vi "LV-Term UI.vi"(11 "LV-Term App In":refnum<class "LV-Term App.lvclass">) -> (3 "LV-Term App":refnum<class "LV-Term App.lvclass">)   [LabVIEW 2020, in "LV-Term.lvlib" / "LV-Term App.lvclass"]
uses:
  LV-Term App.lvclass
  UI State.ctl
  LV-Term App.lvclass/LV-Term App.ctl
  <vilib>/IlluminatedG/IG Terminal/Key Event Data.ctl
  <vilib>/event_ctls.llb/eventvkey.ctl
  <vilib>/IlluminatedG/IG Terminal/Terminal/Terminal.lvclass
  C:/Program Files (x86)/National Instruments/LabVIEW 2020/vi.lib/IlluminatedG/IG OOPanel/OOPanel/Panel/Panel.lvclass
  <vilib>/IlluminatedG/lv-stream/Connection/Connection.lvclass
  <vilib>/IlluminatedG/IG OOPanel/OOPanel/Manager/Manager.lvclass
  <vilib>/IlluminatedG/IG Terminal/Terminal.lvlib
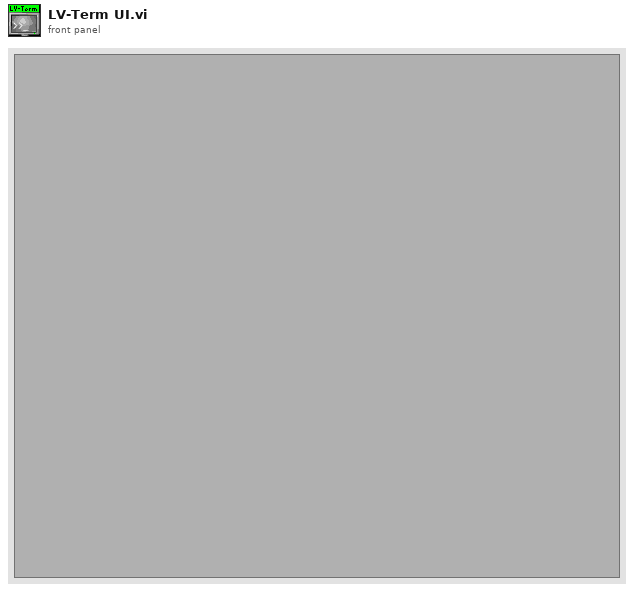
[diagram p1: front panel]
types:
  T1 = typedef "LV-Term.lvlib/LV-Term App.lvclass/UI State.ctl" = enum16{"Init", "Run", "Close"}
  T2 = typedef "Terminal.lvlib/Key Event Data.ctl" = cluster{"Char":i16, "VKey":T3, "ScanCode":i16, "Ctrl":bool}
  T3 = typedef "eventvkey.ctl" = enum16{"ASCII", "Enter", "Return", "Shift", "Ctrl", "Alt", "Cmd", "Opt", "Caps", "NumLock", "Clear", "Break", "Up", "Down", "Left", "Right", "Insert", "Delete", "Home", "End", "PageUp", "PageDown", "Escape", "Help", "Pause", "ScrollLock", "F1", "F2", "F3", "F4", "F5", "F6", "F7", "F8", "F9", "F10", "F11", "F12", "F13", "F14", "F15", "F16", "F17", "F18", "F19", "F20", "F21", "F22", "F23", "F24", "Play", "VolumeUp", "VolumeDown", "Mute", "Two Byte Char"}
  T4 = cluster{"Size Event Reg":refnum<event-registration>}
  T5 = typedef "LVRectTypeDef.ctl" = cluster{"Left":i16, "Top":i16, "Right":i16, "Bottom":i16}
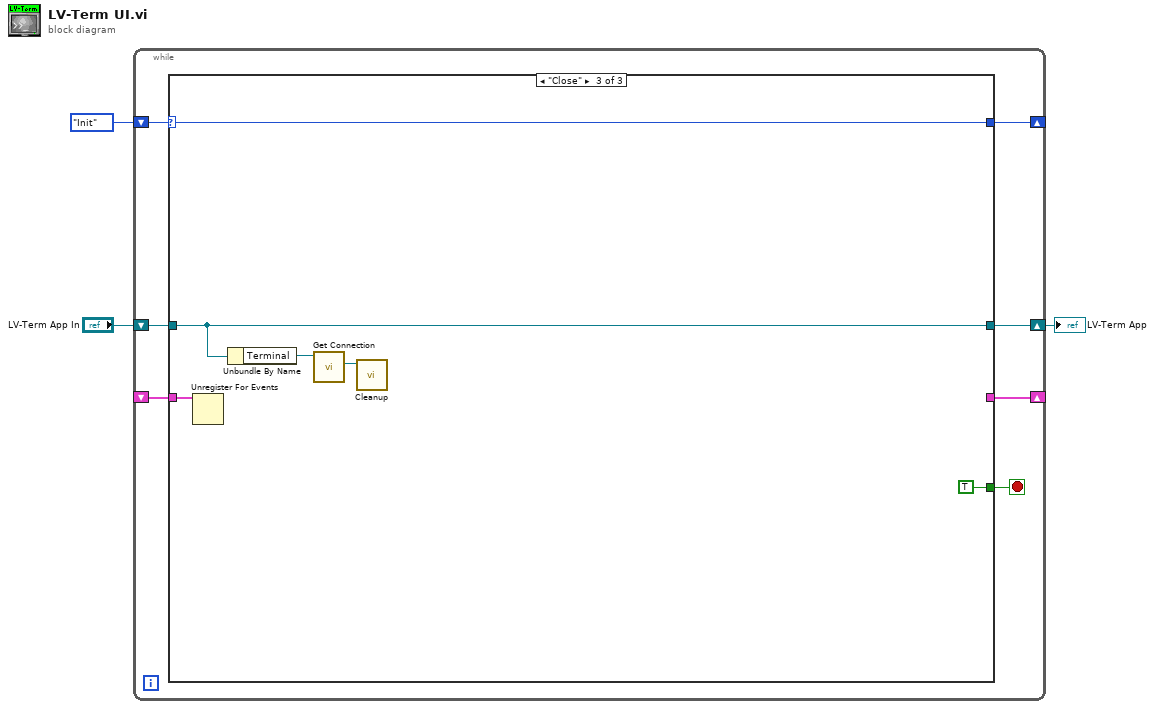
[diagram p0: block diagram]
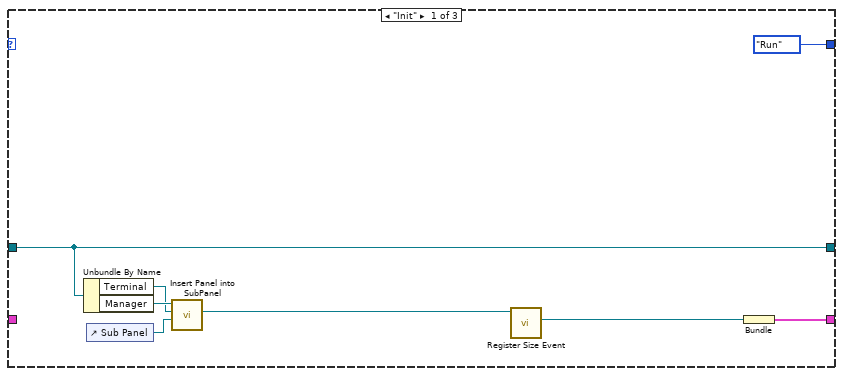
[diagram p2: hidden frame]
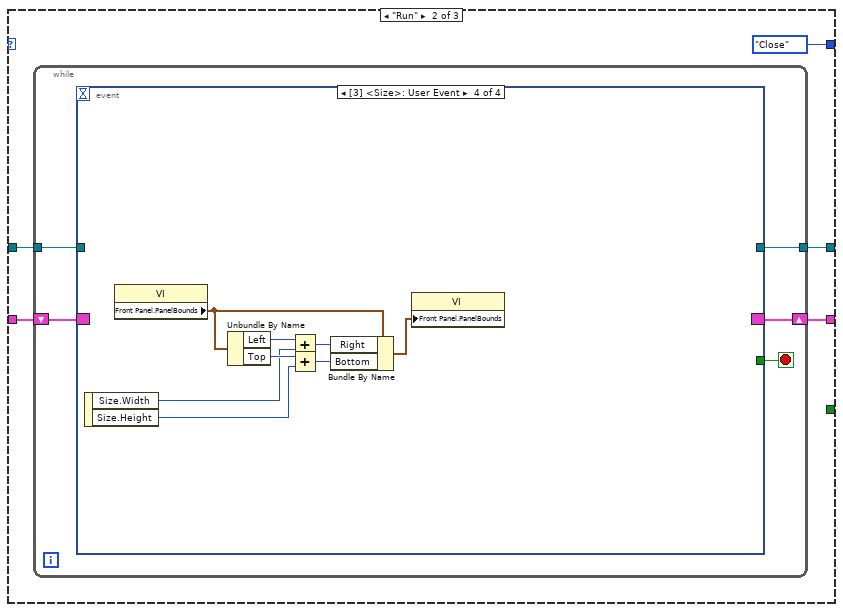
[diagram p3: hidden frame]
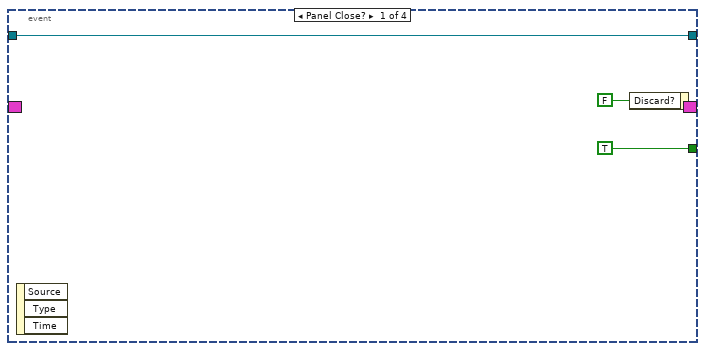
[diagram p4: hidden frame]
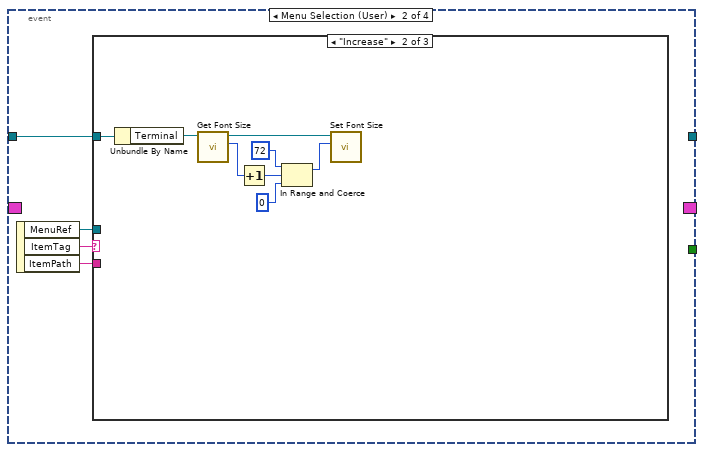
[diagram p5: hidden frame]
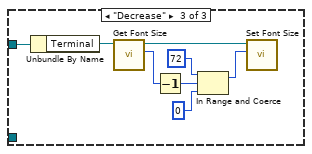
[diagram p7: hidden frame]
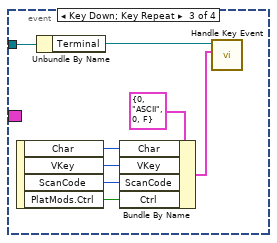
[diagram p8: hidden frame]
diagram:
  n1 = while {
    shift-right: [w9] -> _
    shift-left: UI_State."Init" ("UI State") -> [w10]
    shift-right: [w6] -> w1
    shift-left: "LV-Term App In" -> [w7]
    shift-right: [w5] -> _
    shift-left: _ -> [w4]
    stop <- w8 stop-if-true
    n2 = case shown="\"Close\"" w10 {
      selector: w10 -> [_ _ w72]
      tunnel: [UI_State."Run" ("UI State") UI_State."Close" ("UI State") w72] -> w9
      tunnel: [_ _ TRUE] -> w8
      tunnel: w7 -> [w16 w22 w71]
      tunnel: [w16 w21 w71] -> w6
      tunnel: [w11 w19 _] -> w5
      tunnel: w4 -> [_ w20 w68]
      frame "Init" {
        n3 = Unbundle By Name(w16) -> ("Terminal"=w14:refnum<class "Terminal.lvclass">, "Manager"=w15:refnum<class "Manager.lvclass">)
        n4 = control-ref of="Sub Panel"() -> (w17:refnum<vi>)
        n5 = call <vilib>:"Insert Panel into SubPanel.vi"("SubPanel"=w17, "Panel In"=w14, "Manager in"=w15) -> ("Panel"=w13:refnum<class "Terminal.lvclass">)  [unwired: 6 in, 2 out]
        n6 = call <vilib>:"Register Size Event.vi"("Terminal in"=w13) -> ("Size Event Reg"=w12:refnum<event-registration>)  [unwired: 8 in, 2 out]
        n7 = Bundle("Size Event Reg"=w12) -> (w11:T4)  [unwired: 1 in]
      }
      frame "Run" {
        n8 = while {
          tunnel: w22 -> [w27]
          tunnel: [w26] -> w21
          shift-right: [w24] -> w19
          shift-left: w20 -> [w25]
          stop <- w28 stop-if-true
          n9 = event shown="[3] <Size>: User Event" {
            selector: w25 -> [_ _ _ _]
            dyn-events: [_ _ _ _] -> w24
            timeout: _ -> [_ _ _ _]
            tunnel: [TRUE ("Discard?") _ _ _] -> w28
            tunnel: w27 -> [w29 w32 w59 _]
            tunnel: [w29 _ _ _] -> w26
            event Panel Close? {
              n10 = event-data() -> ()  [unwired: 1 in, 3 out]
              n11 = event-data("Discard?"=FALSE) -> ()  [unwired: 1 in, 1 out]
            }
            event Menu Selection (User) {
              n12 = event-data() -> ("MenuRef"=w34:refnum<k9>, "ItemTag"=w35:string, "ItemPath"=w33:string)  [unwired: 1 in]
              n13 = case shown="\"Increase\"" w35 {
                tunnel: w34 -> [_ _ _]
                tunnel: w33 -> [_ _ _]
                tunnel: w32 -> [_ w36 w51]
                frame Default {
                }
                frame "Increase" {
                  n14 = Unbundle By Name(w36) -> ("Terminal"=w43:refnum<class "Terminal.lvclass">)
                  n15 = call <vilib>:"Get Font Size.vi"("Terminal in"=w43) -> ("Font Size"=w42:i16, "Terminal out"=w38:refnum<class "Terminal.lvclass">)  [unwired: 8 in, 1 out]
                  n16 = Increment(x=w42) -> (x+1=w41:i16)
                  n17 = In Range and Coerce(upper limit=i16 72, x=w41, lower limit=i16 0) -> (coerced(x)=w37:i16)  [unwired: 1 out]
                  n18 = call <vilib>:"Set Font Size.vi"("Font Size"=w37, "Terminal in"=w38) -> ()  [unwired: 8 in, 2 out]
                }
                frame "Decrease" {
                  n19 = Unbundle By Name(w51) -> ("Terminal"=w50:refnum<class "Terminal.lvclass">)
                  n20 = call <vilib>:"Get Font Size.vi"("Terminal in"=w50) -> ("Font Size"=w49:i16, "Terminal out"=w45:refnum<class "Terminal.lvclass">)  [unwired: 8 in, 1 out]
                  n21 = Decrement(x=w49) -> (x-1=w48:i16)
                  n22 = In Range and Coerce(upper limit=i16 72, x=w48, lower limit=i16 0) -> (coerced(x)=w44:i16)  [unwired: 1 out]
                  n23 = call <vilib>:"Set Font Size.vi"("Font Size"=w44, "Terminal in"=w45) -> ()  [unwired: 8 in, 2 out]
                }
              }
            }
            event Key Down; Key Repeat {
              n24 = event-data() -> ("Char"=w55:i16, "VKey"=w54:T3, "ScanCode"=w53:i16, "PlatMods.Ctrl"=w52:bool)  [unwired: 1 in]
              n25 = Unbundle By Name(w59) -> ("Terminal"=w58:refnum<class "Terminal.lvclass">)
              n26 = Bundle By Name(cluster=T2 {"Char"=0, "VKey"=enum."ASCII", "ScanCode"=0, "Ctrl"=FALSE} ("Key Event Data"), "Char"=w55, "VKey"=w54, "ScanCode"=w53, "Ctrl"=w52) -> (w56:T2)
              n27 = call <vilib>:"Handle Key Event.vi"("Key Event Data"=w56, "Terminal in"=w58) -> ()  [unwired: 8 in, 2 out]
            }
            event User Event {
              n28 = event-data() -> ("Size.Width"=w65:u32, "Size.Height"=w64:u32)  [unwired: 1 in]
              n29 = property class="VI"() -> ("Front Panel.PanelBounds"=w63:T5)  [unwired: 2 in, 2 out]
              n30 = Unbundle By Name(w63) -> ("Left"=w66:i16, "Top"=w67:i16)
              n31 = Add(x=w66, y=w65) -> (x+y=w62:u32)
              n32 = Add(x=w67, y=w64) -> (x+y=w61:u32)
              n33 = Bundle By Name(cluster=w63, "Right"=w62, "Bottom"=w61) -> (w60:T5)
              n34 = property class="VI"("Front Panel.PanelBounds"=w60) -> ()  [unwired: 2 in, 2 out]
            }
          }
        }
      }
      frame "Close" {
        n35 = Unregister For Events(event registration refnum=w68) -> ()  [unwired: 1 in, 1 out]
        n36 = Unbundle By Name(w71) -> ("Terminal"=w70:refnum<class "Terminal.lvclass">)
        n37 = call <vilib>:"Get Connection.vi"("Terminal in"=w70) -> ("Connection"=w69:refnum<class "Connection.lvclass">)  [unwired: 8 in, 2 out]
        n38 = call-dynamic "Cleanup.vi"("Connection in"=w69) -> ()  [unwired: 10 in, 1 out]
      }
    }
  }
  "LV-Term App" <- w1
